vi "Ex-03 Acq Finite Multipoint & FFT.vi"() -> ()   [LabVIEW 2012]
doc: "© Copyright M. Ferrari 2012\nMultipoint Analog Acq. Mean & FFT"
uses:
  <vilib>/DAQmx/create/channels.llb/DAQmx Create Channel (AI-Voltage-Basic).vi
  <vilib>/DAQmx/configure/timing.llb/DAQmx Timing (Sample Clock).vi
  <vilib>/DAQmx/read.llb/DAQmx Read (Analog Wfm 1Chan NSamp).vi
  <vilib>/express/express analysis/Spectral/XNode/ExpressSpectralMeasurementsBlockNode.xnode
  <vilib>/express/express analysis/Spectral/Block/exnSpectralBlock spectral measurements RMS poly.vi
  <vilib>/express/express analysis/Spectral/Block/exnSpectralBlock spectral measurements RMS WFM.vi
  <vilib>/measure/NI_MAPro.lvlib
  <vilib>/measure/maspectr.llb/FFT Spectrum (Mag-Phase) for 1 Chan.vi
  <vilib>/measure/NI_MABase.lvlib
panel:
  in  "Ampiezza\ndi rumore":dbl=1.0 format="%.2p"
  in  "n° samples":i32=1000
  in  "rate":dbl=10000.0
  in  "min":dbl=-5.0 format="%0.2f"
  in  "max":dbl=5.0 format="%0.2f"
  in  "in conf":i32(ring)=10083 items=["default"=-1, "RSE"=10083, "NRSE"=10078, "Differential"=10106, "Pseudodifferential"=12529]
  in  "physical ch":tag="Dev1/ai0"
  out "FFT":cluster{"f0":dbl, "df":dbl, "magnitude":dbl[]}(graph)
  out "FFT - (RMS)":cluster{"f0":dbl, "df":dbl, "magnitude":dbl[]}
  out "Volt Graph":waveform(dbl)(graph)
  out "mean":dbl format="%0.2f"
  # "RANGE"
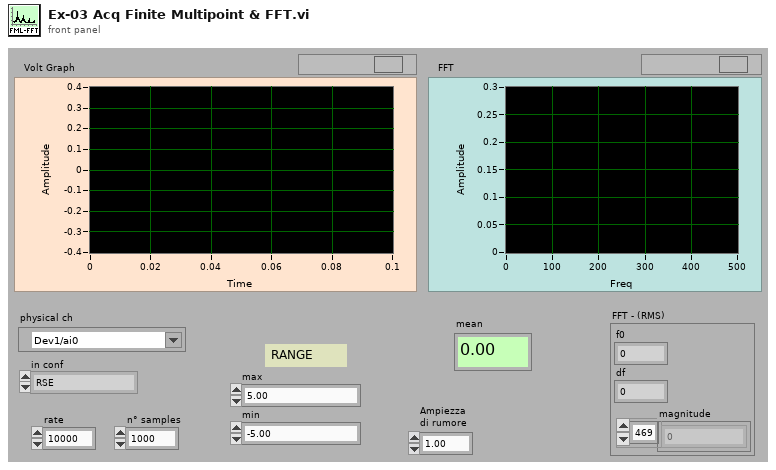
[diagram p1: front panel]
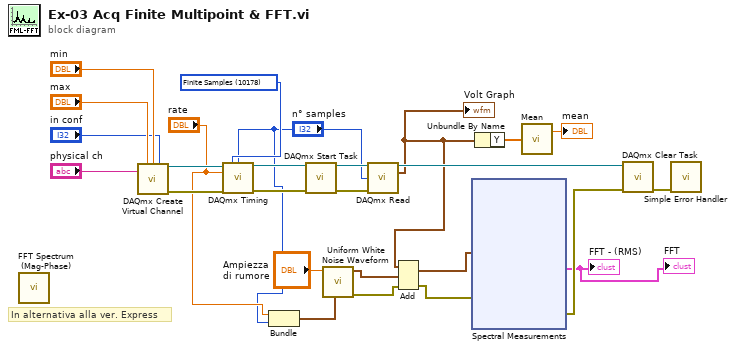
[diagram p0: block diagram]
diagram:
  w22 = 10178 items=["Finite Samples"=10178, "Continuous Samples"=10123, "Hardware Timed Single Point"=12522] ("sample mode")
  # "In alternativa alla ver. Express"
  n1 = call-poly <vilib>:"FFT Spectrum (Mag-Phase).vi"() -> ()  [unwired: 7 in, 5 out]
  n2 = call-poly <vilib>:"DAQmx Create Virtual Channel.vi"("maximum value"="max", "minimum value"="min", "input terminal configuration"="in conf", "physical channels"="physical ch") -> ("task out"=w21:refnum<k21>, "error out"=w20:errorcluster)  [unwired: 5 in, 5 out]
  n3 = call-poly <vilib>:"DAQmx Timing.vi"("task/channels in"=w21, "sample mode"=w22, "samples per channel"="n° samples", "rate"="rate", "error in"=w20) -> ("task out"=w19:refnum<k21>, "error out"=w18:errorcluster)  [unwired: 2 in, 7 out]
  n4 = Bundle("rate"="rate", "n° samples"="n° samples") -> (w5:cluster{"rate":dbl, "n° samples":i32})  [unwired: 1 in]
  n5 = call <vilib>:"DAQmx Start Task.vi"("task/channels in"=w19, "error in"=w18) -> ("task out"=w17:refnum<k21>, "error out"=w16:errorcluster)  [unwired: 12 out]
  n6 = call <vilib>:"Uniform White Noise Waveform.vi"("sampling info"=w5, "amplitude"="Ampiezza\ndi rumore") -> ("error out"=w6:errorcluster, "signal out"=w8:waveform(dbl))  [unwired: 8 in]
  n7 = call-poly <vilib>:"DAQmx Read.vi"("task/channels in"=w17, "number of samples per channel"="n° samples", "error in"=w16) -> ("task out"=w13:refnum<k21>, "data"=w9:waveform(dbl))  [unwired: 11 out]
  "Volt Graph" <- w9
  n8 = Add(1:w8, 2:w9, 4:w6) -> (0:w10:waveform(dbl), 3:w7:errorcluster)
  n9 = xnode "Spectral Measurements"("Signals"=w10, "error in (no error)"=w7) -> ("FFT - (RMS)"=→"FFT - (RMS)" →"FFT":cluster{"f0":dbl, "df":dbl, "magnitude":dbl[]}, "error out"=w12:errorcluster)  [unwired: 1 out]
  n10 = Unbundle By Name(w9) -> ("Y"=w15:dbl[])
  n11 = call <vilib>:"Mean.vi"("X"=w15) -> ("mean"=→"mean":dbl)  [unwired: 1 out]
  n12 = call <vilib>:"DAQmx Clear Task.vi"("task in"=w13, "error in"=w12) -> ("error out"=w11:errorcluster)  [unwired: 13 out]
  n13 = call <vilib>:"Simple Error Handler.vi"("error in (no error)"=w11) -> ()  [unwired: 1 in, 8 out]
